vi "(SubVI)Serial_Read.vi"(5 "Checksum Verification":bool, 7 "Header Verification":bool, 8 "error in (no error)":errorcluster caption="에러 입력(에러 없음)", 11 "Function":T1=enum."Read") -> (0 "error out":errorcluster caption="에러 출력", 2 "Header":T2 {"Delimiter Code" format="%02x"; "BD Info" format="%02x"; "Msg Size" format="%04x"; "Checksum" format="%02x"; "Echo Request" format="%02x"}, 3 "Read Data":u8[](array[numeric]))   [LabVIEW 2020]
uses:
  Controls/(Ctrl)Serial_Protocol Header.ctl
  Controls/(Ctrl)Serial_FGV Function.ctl
  Variables/(Var)System Variables.vi
panel:
  # "(SubVI)Serial_Read.vi By hspark\n\nDescription : 시리얼 통신으로 Header와 Data를 읽는 VI\n\nInput : \n1. Header Verification : True 입력 시 Header에서 구분자 코드, 보드 정보를 검증함\n2. Checksum Verification : True 입력 시 Header의 Checksum 값과 읽은 Data의 Checksum 연산 값을 검증함\n\nOutput : \n1. Read Data : 읽은 Data를 U8 배열로 변환하여 출력\n2. Header : 읽은 Header를 클러스터로 출력\n\nLabVIEW Version : 2020 SP1 이상\n\nNote :\n\nUpdate : 2021.10.06"
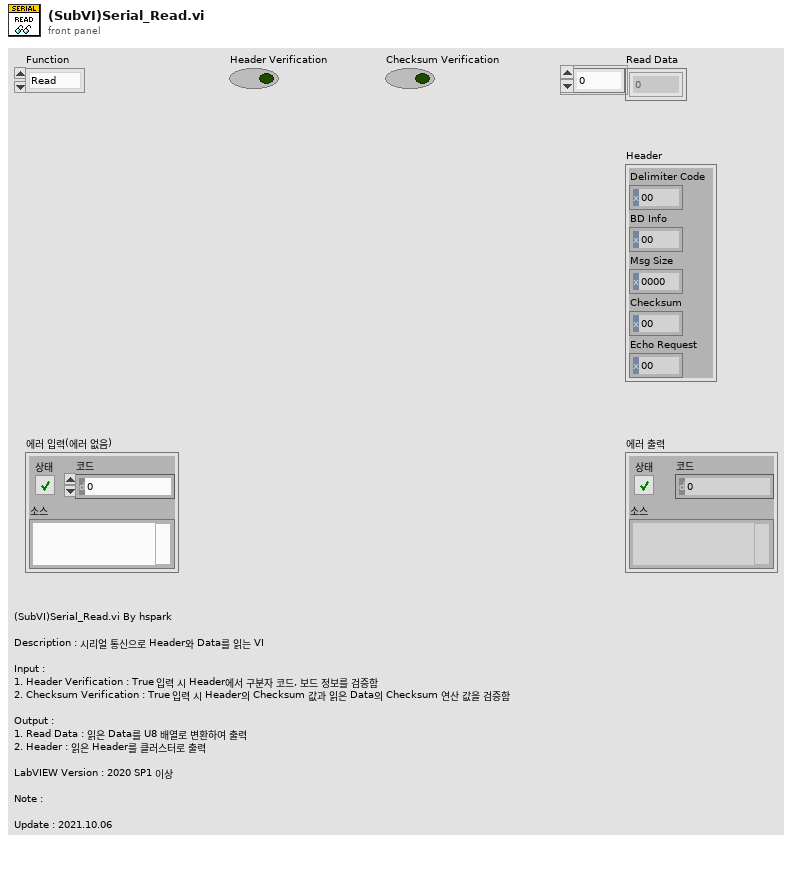
[diagram p1: front panel]
types:
  T1 = typedef "(Ctrl)Serial_FGV Function.ctl" = enum16{"Initialize", "Read", "Read All", "Write", "Flush Buffer", "Get Ref.", "Close"}
  T2 = typedef "(Ctrl)Serial_Protocol Header.ctl" = cluster{"Delimiter Code":u8, "BD Info":u8, "Msg Size":u16, "Checksum":u8, "Echo Request":u8}
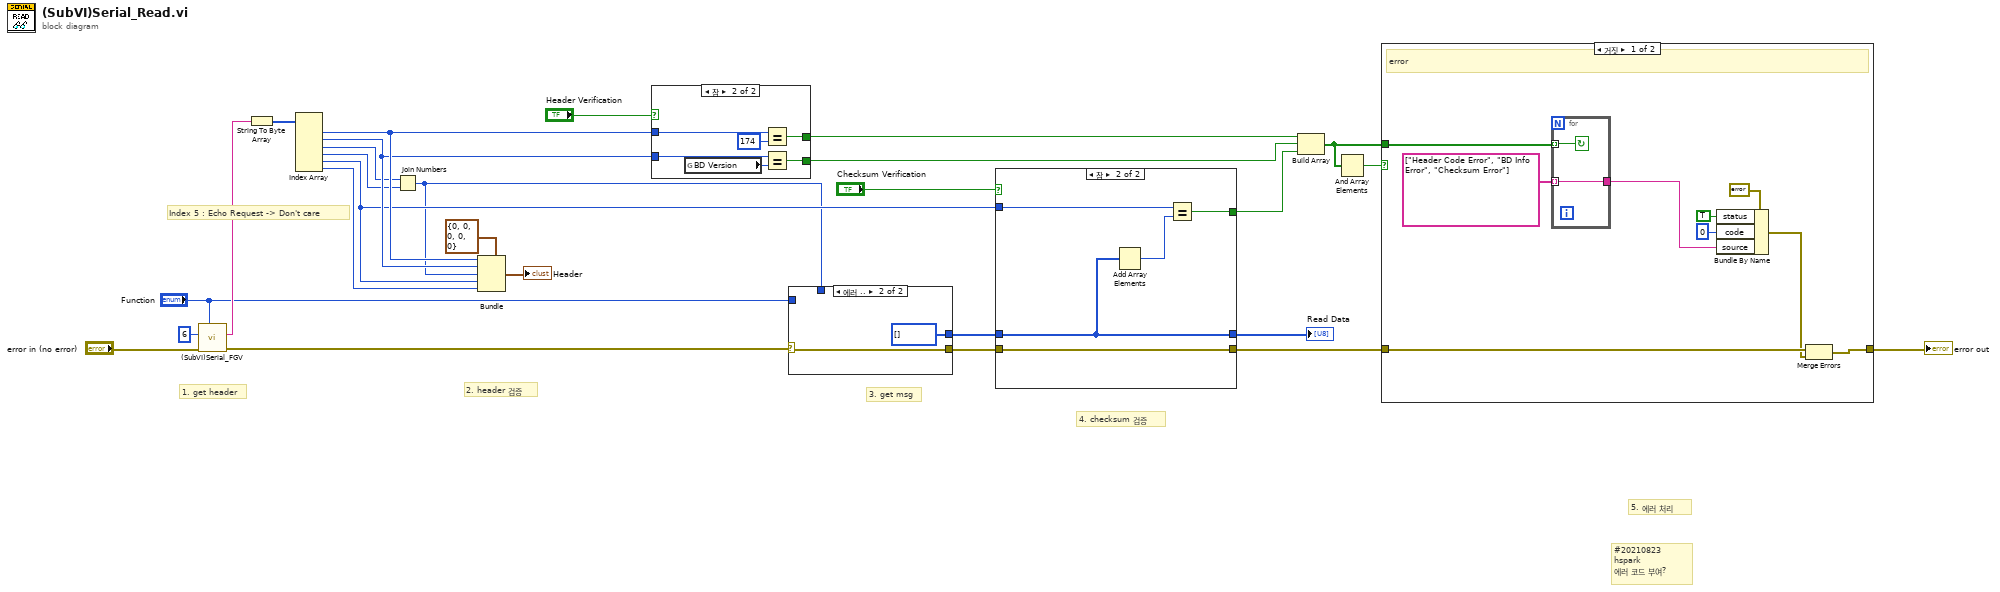
[diagram p0: block diagram]
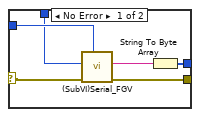
[diagram p2: hidden frame]
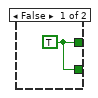
[diagram p4: hidden frame]
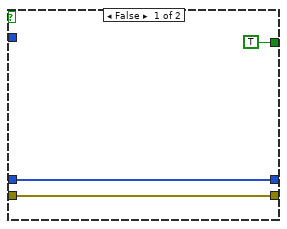
[diagram p5: hidden frame]
diagram:
  # "#20210823\nhspark\n에러 코드 부여?"
  # "5. 에러 처리"
  # "4. checksum 검증"
  # "2. header 검증"
  # "3. get msg"
  # "1. get header"
  # "Index 5 : Echo Request -> Don't care"
  n1 = call "(SubVI)Serial_FGV.vi"("Function"="Function", "error in (no error)"="error in (no error)", "Bytes to Read"=u32 6) -> ("error out"=w1:errorcluster, "Read Data"=w25:string)  [unwired: 6 in, 1 out]
  n2 = String To Byte Array(string=w25) -> (unsigned byte array=w24:u8[])
  n3 = Index Array(array=w24) -> (element #1=w15:u8, element #2=w14:u8, element #3=w13:u8, element #4=w12:u8, element #5=w9:u8, element #6=w8:u8)  [unwired: 6 in]
  n4 = Join Numbers(hi=w13, lo=w12) -> ((hi.lo)=w3:u16)
  n5 = Bundle(cluster=T2 {"Delimiter Code"=0, "BD Info"=0, "Msg Size"=0, "Checksum"=0, "Echo Request"=0} ("클러스터"), "Delimiter Code"=w15, "BD Info"=w14, "Msg Size"=w3, "Checksum"=w9, "Echo Request"=w8) -> (→"Header":T2)
  n6 = case shown="참" "Header Verification" {
    tunnel: w15 -> [_ w34]
    tunnel: w14 -> [_ w32]
    tunnel: [w28 w30] -> w21
    tunnel: [w28 w29] -> w20
    frame False {
      w28 = TRUE
    }
    frame True {
      n7 = global read "(Var)System Variables.vi" "BD Version"() -> (w31:u8)
      n8 = Equal?(x=w34, y=u8 174) -> (x = y?=w30:bool)
      n9 = Equal?(x=w32, y=w31) -> (x = y?=w29:bool)
    }
  }
  n10 = case shown="에러 .." w1 {
    selector: w1 -> [w35 w42]
    tunnel: [w39 u8[] [] ("unsigned byte array")] -> w5
    tunnel: "Function" -> [w38 _]
    tunnel: w3 -> [w37 _]
    tunnel: [w36 w42] -> w2
    frame No Error {
      n11 = call "(SubVI)Serial_FGV.vi"("Function"=w38, "error in (no error)"=w35, "Bytes to Read"=w37) -> ("error out"=w36:errorcluster, "Read Data"=w40:string)  [unwired: 6 in, 1 out]
      n12 = String To Byte Array(string=w40) -> (unsigned byte array=w39:u8[])
    }
    frame Error {
    }
  }
  n13 = case shown="참" "Checksum Verification" {
    tunnel: w5 -> [w44 w46]
    tunnel: w9 -> [_ w49]
    tunnel: w2 -> [w45 w48]
    tunnel: [w45 w48] -> w6
    tunnel: [w44 w46] -> w7
    tunnel: [TRUE w47] -> w19
    frame False {
    }
    frame True {
      n14 = Add Array Elements(numeric array=w46) -> (sum=w50:u8)
      n15 = Equal?(x=w49, y=w50) -> (x = y?=w47:bool)
    }
  }
  "Read Data" <- w7
  n16 = Build Array(w21, w20, w19) -> (w16:bool[])
  n17 = And Array Elements(Boolean array=w16) -> (logical AND=w17:bool)
  n18 = case shown="거짓" w17 {
    tunnel: w6 -> [w56 w62]
    tunnel: [w55 w62] -> w22
    tunnel: w16 -> [w51 _]
    frame False {
      # "error"
      n19 = for {
        tunnel: w51 -> [w60] mode=indexing
        tunnel: string[] ["Header Code Error", "BD Info Error", "Checksum Error"] -> [w61] mode=indexing
        tunnel: [w61] -> w52
        stop <- w60 continue-if-true
      }
      n20 = Bundle By Name(cluster=errorcluster {"status"=FALSE, "code"=0, "source"=""} ("error out"), "status"=TRUE, "code"=0, "source"=w52) -> (w53:errorcluster)
      n21 = Merge Errors(w56, w53) -> (w55:errorcluster)
    }
    frame True {
      # "no error"
    }
  }
  "error out" <- w22
